vi "Write TxPkt Thread Sync.vi"(8 "error in (no error)":errorcluster, 10 "threadSync":T1 caption="Synchronization", 11 "Node Ptr":T2 format="%.0x") -> (0 "error out":errorcluster, 3 "Node Ptr out":T2 format="%.0x")   [LabVIEW 2019, in "UDP-Custom-Device System Explorer.lvlib" / "Tx Packet Accessors.lvlib"]
uses:
  Tx Packet Accessors.lvlib
  <vilib>/NI VeriStand/Custom Device API/Custom Device Item Ref.ctl
  Types/Threading/Thread Sync Reference.ctl
  Shared/Constants.vi
  <vilib>/NI VeriStand/Custom Device API/Set Item Property (U16).vi
  <vilib>/NI VeriStand/Custom Device API/Custom Device API.lvlib
  Shared/UDP-Custom-Device Shared.lvlib
  UDP-Custom-Device System Explorer.lvlib
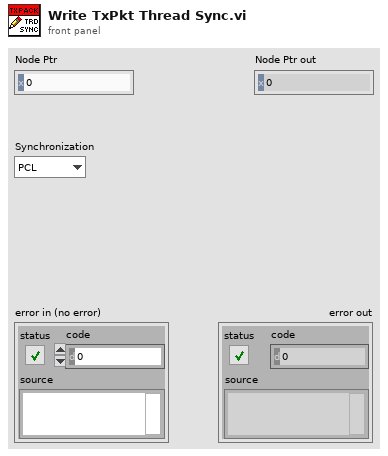
[diagram p1: front panel]
types:
  T1 = typedef "UDP-Custom-Device System Explorer.lvlib/Thread Sync Reference.ctl" = enum16{"PCL", "Async"}
  T2 = typedef "Custom Device API.lvlib/Custom Device Item Ref.ctl" = u64
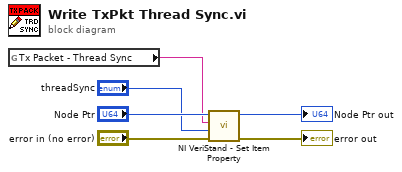
[diagram p0: block diagram]
diagram:
  n1 = global read "Constants.vi" "Tx Packet - Thread Sync"() -> (w1:string)
  n2 = call-poly <vilib>:"NI VeriStand - Set Item Property.vi"("error in (no error)"="error in (no error)", "Value"="threadSync", "Property Name"=w1, "Item Ref in"="Node Ptr") -> ("error out"=→"error out":errorcluster, "Item Ref out"=→"Node Ptr out":T2)  [unwired: 5 in, 1 out]
